vi "save data.vi"(7 "experiment name":string="01_90_01", 9 "packet number":u32=30, 10 "?":bool=TRUE, 11 "samples":cdb[](array[numeric])) -> (0 "error out":errorcluster, 1 "Done":bool=TRUE, 2 "packets in buf (%)":dbl(slide)=1000.0 scale=0.0..1.0, 3 "packet number in buf":u32=30, 4 "samples string buffer":string)   [LabVIEW 2020]
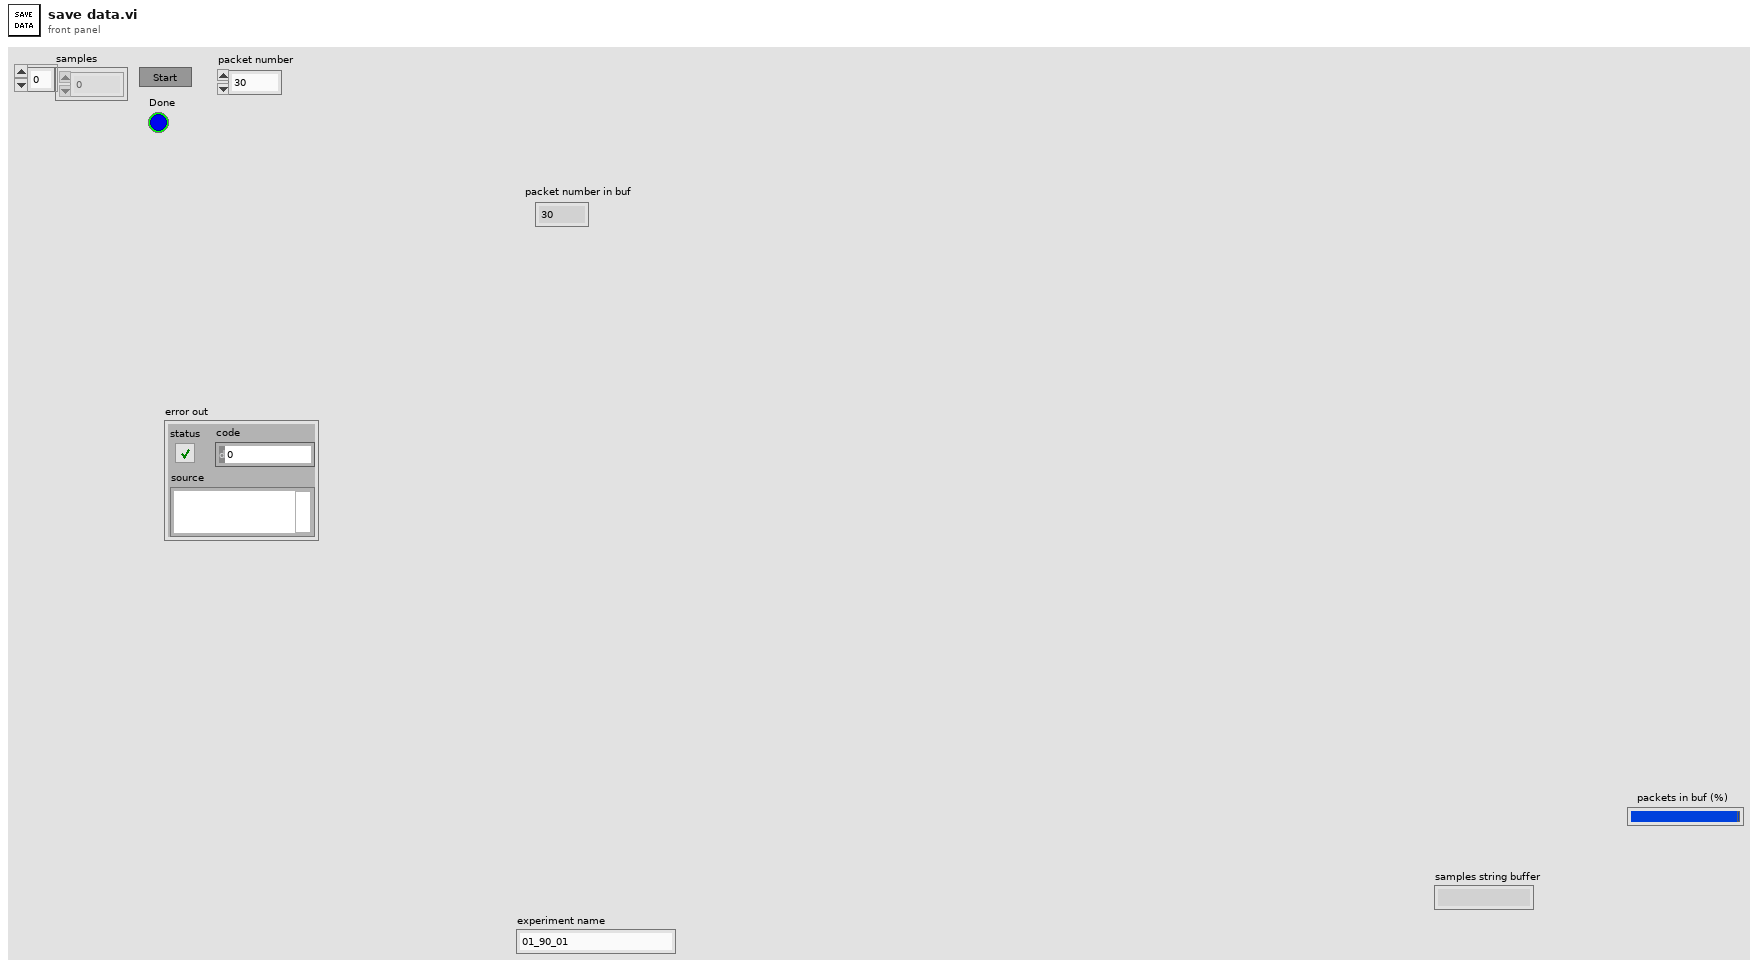
[diagram p1: front panel]
types:
  T1 = enum16{"open", "replace", "create", "open or create", "replace or create", "replace or create with confirmation"}
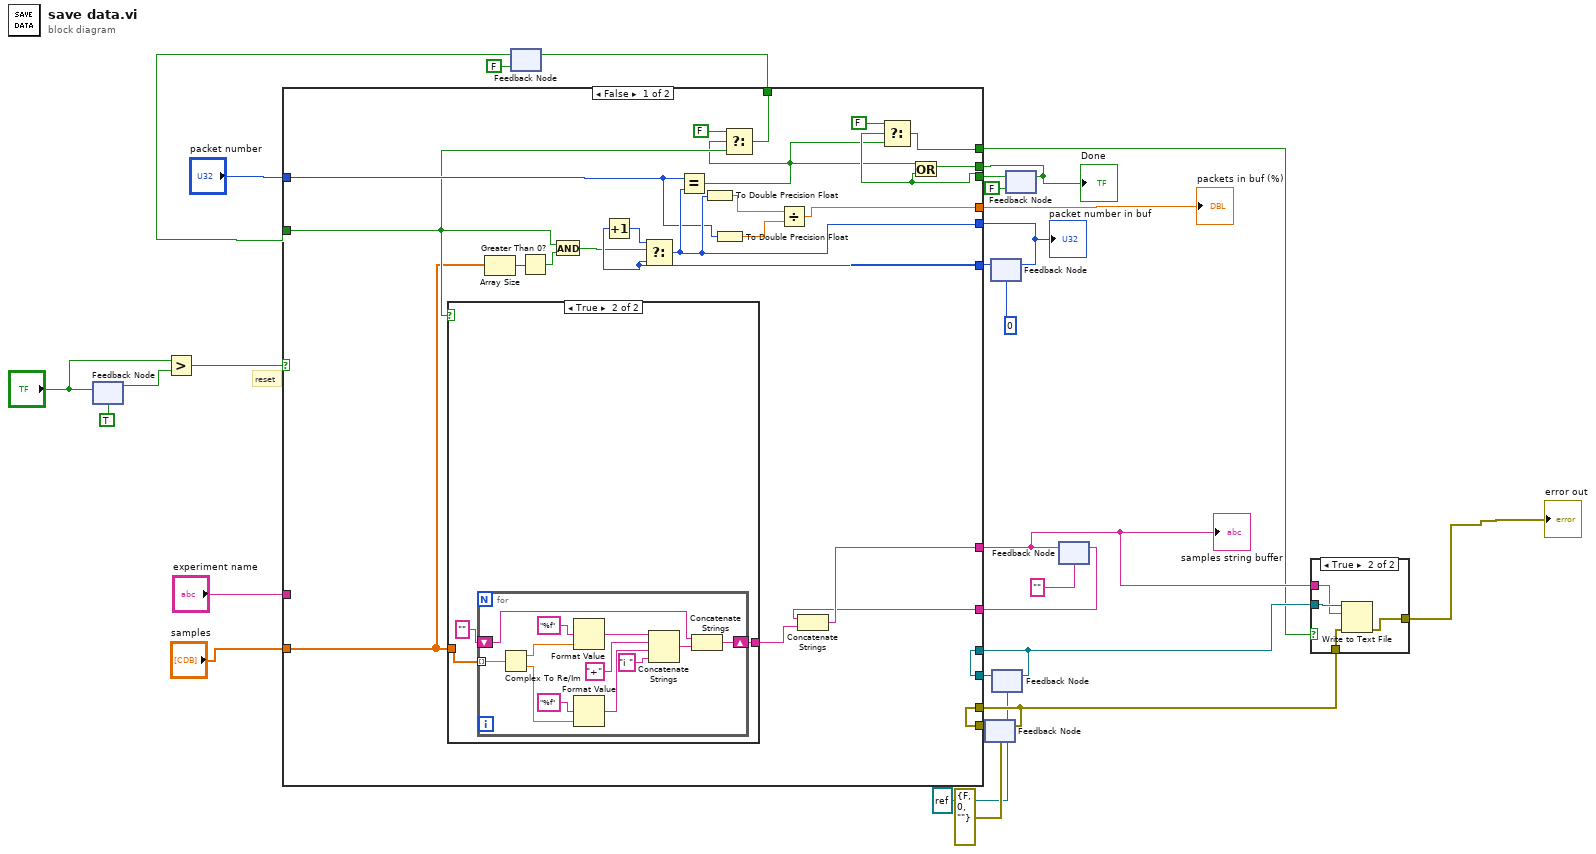
[diagram p0: block diagram]
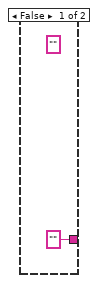
[diagram p3: hidden frame]
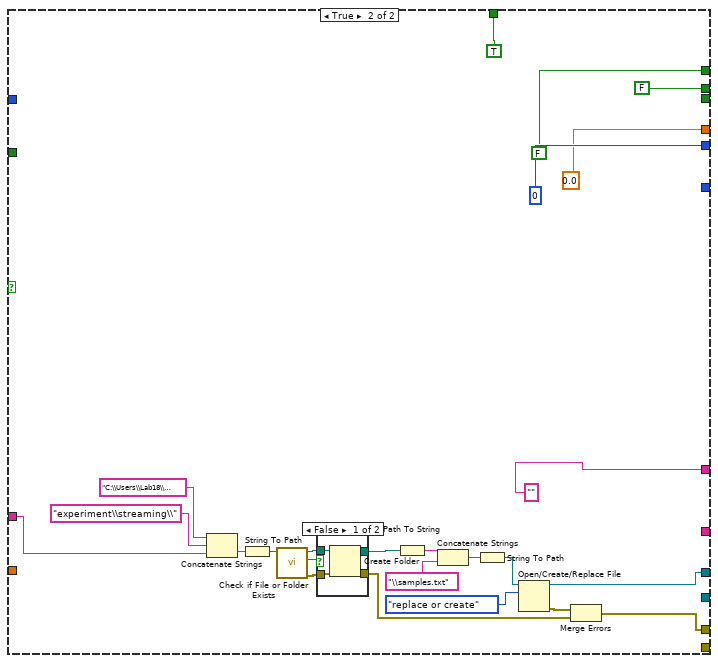
[diagram p4: hidden frame]
diagram:
  # "reset"
  n1 = feedback #1(TRUE) -> (w27:bool)
  n2 = feedback-in #1("?") -> ()
  n3 = Greater?(x="?", y=w27) -> (0:w24:bool)
  n4 = feedback #2(FALSE ("t")) -> (w9:bool)
  n5 = feedback #3(errorcluster {"status"=FALSE, "code"=0, "source"=""} ("error out")) -> (w20:errorcluster)
  n6 = feedback #4(u32 0 ("packet number in buf")) -> (w16:u32)
  n7 = feedback #5(refnum<file> refnum ("samples file")) -> (w21:refnum<file>)
  n8 = feedback #6(FALSE) -> (w8:bool)
  n9 = feedback #7("" ("output string")) -> (w12:string)
  n10 = case shown="False" w24 {
    tunnel: "experiment name" -> [_ w71]
    tunnel: [w51 w70] -> w22
    tunnel: w21 -> [w51 _]
    tunnel: [w30 w69] -> w19
    tunnel: w20 -> [w30 _]
    tunnel: "samples" -> [w29 _]
    tunnel: [w45 u32 0 ("packet number in buf")] -> w17
    tunnel: w9 -> [w37 _]
    tunnel: w16 -> [w49 _]
    tunnel: "packet number" -> [w44 _]
    tunnel: [w32 FALSE] -> w11
    tunnel: [w46 0.0] -> w14
    tunnel: [w43 ""] -> w13
    tunnel: w12 -> [w42 _]
    tunnel: [w38 TRUE] -> w10
    tunnel: [w35 FALSE] -> w7
    tunnel: w8 -> [w34 _]
    frame False {
      n11 = case shown="True" w37 {
        tunnel: ["" w55] -> w52
        tunnel: w29 -> [_ w54]
        frame False {
          (unwired) ""
        }
        frame True {
          n12 = for {
            shift-right: [w67] -> w55
            shift-left: "" -> [w68]
            tunnel: w54 -> [w57] mode=indexing
            n13 = Complex To Re/Im(x + iy=w57) -> (x=w59:dbl, y=w58:dbl)
            n14 = Format Value(format string="%f", value (0)=w59) -> (output string=w66:string)  [unwired: 1 in]
            n15 = Format Value(format string="%f", value (0)=w58) -> (output string=w65:string)  [unwired: 1 in]
            n16 = Concatenate Strings(w66, "+" ("string"), w65, "i " ("string")) -> (w60:string)
            n17 = Concatenate Strings(w68, w60) -> (w67:string)
          }
        }
      }
      n18 = Array Size(array=w29) -> (size(s)=w41:i32)
      n19 = Greater Than 0?(x=w41) -> (x > 0?=w40:bool)
      n20 = And(x=w37, y=w40) -> (x .and. y?=w39:bool)
      n21 = Increment(x=w49) -> (x+1=w50:u32)
      n22 = Select(t=w50, s=w39, f=w49) -> (s? t:f=w45:u32)
      n23 = Equal?(x=w44, y=w45) -> (x = y?=w33:bool)
      n24 = To Double Precision Float(number=w45) -> (double precision float=w48:dbl)
      n25 = To Double Precision Float(number=w44) -> (double precision float=w47:dbl)
      n26 = Select(t=FALSE, s=w33, f=w37) -> (s? t:f=w38:bool)
      n27 = Divide(x=w48, y=w47) -> (x/y=w46:dbl)
      n28 = Concatenate Strings(w42, w52) -> (w43:string)
      n29 = Select(t=FALSE, s=w34, f=w33) -> (s? t:f=w32:bool)
      n30 = Or(x=w33, y=w34) -> (x .or. y?=w35:bool)
    }
    frame True {
      n31 = Concatenate Strings("C:\\Users\\Lab18\\Documents\\LabVIEW Data\\4-х каналка\\", "experiment\\streaming\\", w71) -> (w79:string)
      n32 = String To Path(string=w79) -> (path=w82:path)
      n33 = call <vilib>:"Check if File or Folder Exists.vi"("path"=w82) -> ("error out"=w84:errorcluster, "file or folder exists?"=w85:bool, "dup path"=w83:path)  [unwired: 8 in]
      n34 = case shown="False" w85 {
        tunnel: [w96 w97] -> w78
        tunnel: [w95 w98] -> w80
        tunnel: w83 -> [w94 w97]
        tunnel: w84 -> [w93 w98]
        frame False {
          n35 = Create Folder(path (use dialog)=w94, error in=w93) -> (created path=w96:path, error out=w95:errorcluster)  [unwired: 1 in, 1 out]
        }
        frame True {
        }
      }
      n36 = Path To String(path=w78) -> (string=w86:string)
      n37 = Concatenate Strings(w86, "\\samples.txt") -> (w76:string)
      n38 = String To Path(string=w76) -> (path=w77:path)
      n39 = Open/Create/Replace File(file path (use dialog)=w77, operation (0:open)=T1."replace or create") -> (refnum out=w70:refnum<file>, error out=w81:errorcluster)  [unwired: 4 in, 1 out]
      n40 = Merge Errors(w81, w80) -> (w69:errorcluster)
    }
  }
  "Done" <- w7
  "samples string buffer" <- w13
  "packet number in buf" <- w17
  "packets in buf (%)" <- w14
  n41 = feedback-in #2(w10) -> ()
  n42 = feedback-in #3(w19) -> ()
  n43 = feedback-in #4(w17) -> ()
  n44 = feedback-in #5(w22) -> ()
  n45 = feedback-in #6(w7) -> ()
  n46 = feedback-in #7(w13) -> ()
  n47 = case shown="True" w11 {
    tunnel: w22 -> [_ w103]
    tunnel: w13 -> [_ w102]
    tunnel: [w99 w101] -> w1
    tunnel: w19 -> [w99 w100]
    frame False {
    }
    frame True {
      n48 = Write to Text File(file (use dialog)=w103, text=w102, error in=w100) -> (error out=w101:errorcluster)  [unwired: 1 in, 2 out]
    }
  }
  "error out" <- w1
